vi "ke37xx Simple Measurement Example.vi"() -> ()   [LabVIEW 2009]
doc: "Simple Measurement Example\n \nThis sample shows very basic measurement operations performed\nwith the Ke37XX. The measurement function is selectable, as is\nthe number of times the specified measurement should be performed.\nThe results of each operation are presented in the results\nlistbox control."
uses:
  <instrlib>/Keithley 3706/Keithley 3700 Series.lvlib
panel:
  in  "Measure Count (10)":u32=10 min=1
  in  "Function (2: DC Volts)":T1(ring)=enum."DC Volts"
  out "Measurements":dbl[](array[numeric]) format="%#_6e"
  in  "VISA Resource Name":refnum<visa-resource-name>="GPIB::6"
  in  "Timeout (30000 milliseconds)":u32=30000
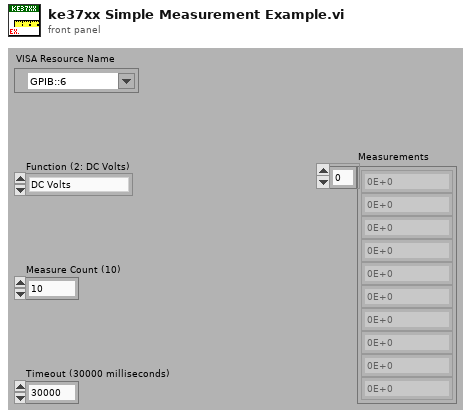
[diagram p1: front panel]
types:
  T1 = enum16{"None", "DC Volts", "AC Volts", "DC Current", "AC Current", "2-Wire Ohms", "4-Wire Ohms", "Temperature", "Period", "Frequency", "Continuity", "Commonside Ohms"}
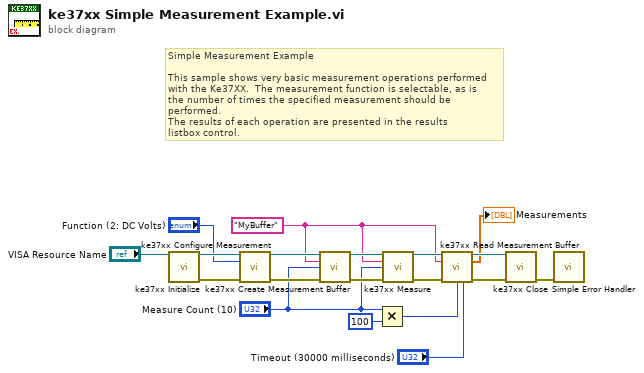
[diagram p0: block diagram]
diagram:
  w7 = "MyBuffer" ("Buffer Name")
  # "Simple Measurement Example\n \nThis sample shows very basic measurement operations performed\nwith the Ke37XX.  The measurement function is selectable, as is\nthe number of times the specified measurement should be performed.\nThe results of each operation are presented in the results\nlistbox control."
  n1 = call <instrlib>:"ke37xx Initialize.vi"("VISA resource name"="VISA Resource Name") -> ("VISA resource name out"=w18:refnum<visa-resource-name>, "error out"=w14:errorcluster)  [unwired: 13 in]
  n2 = call <instrlib>:"ke37xx Configure Measurement.vi"("VISA Resource Name"=w18, "Function (0: None)"="Function (2: DC Volts)", "error in (no error)"=w14) -> ("VISA Resource Name Out"=w13:refnum<visa-resource-name>, "error out"=w12:errorcluster)  [unwired: 11 in]
  n3 = call <instrlib>:"ke37xx Create Measurement Buffer.vi"("VISA Resource Name"=w13, "Buffer Name"=w7, "Capacity"="Measure Count (10)", "error in (no error)"=w12) -> ("VISA Resource Name Out"=w11:refnum<visa-resource-name>, "error out"=w10:errorcluster)  [unwired: 10 in]
  n4 = Multiply(x="Measure Count (10)", y=u32 100) -> (x*y=w2:u32)
  n5 = call <instrlib>:"ke37xx Measure.vi"("VISA Resource Name"=w11, "Buffer Name"=w7, "Measure Count (1)"="Measure Count (10)", "error in (no error)"=w10) -> ("VISA Resource Name Out"=w9:refnum<visa-resource-name>, "error out"=w8:errorcluster)  [unwired: 7 in, 3 out]
  n6 = call <instrlib>:"ke37xx Read Measurement Buffer.vi"("VISA Resource Name"=w9, "Buffer Name"=w7, "error in (no error)"=w8, "Bytes To Read (1024)"=w2, "Timeout (10 seconds)"="Timeout (30000 milliseconds)") -> ("VISA Resource Name Out"=w19:refnum<visa-resource-name>, "Readings"=→"Measurements":dbl[], "error out"=w3:errorcluster)  [unwired: 4 in, 4 out]
  n7 = call <instrlib>:"ke37xx Close.vi"("VISA resource name"=w19, "error in (no error)"=w3) -> ("error out"=w16:errorcluster)  [unwired: 13 in]
  n8 = call <vilib>:"Simple Error Handler.vi"("error in (no error)"=w16) -> ()  [unwired: 1 in, 8 out]
